vi "azimut.vi"() -> (0 "Numeric":u8)   [LabVIEW 2015, in "Igor.lvclass"]
uses:
  Igor.lvclass
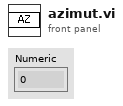
[diagram p1: front panel]
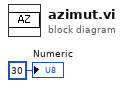
[diagram p0: block diagram]
diagram:
  "Numeric" <- u8 30
